vi "Rotate.vi"(2 "Angle(rad)":dbl format="%.5f", 3 "Y":dbl format="%.2f", 4 "X":dbl format="%.2f") -> (0 "rotY":dbl format="%.5f", 1 "rotX":dbl format="%.5f")   [LabVIEW 2011]
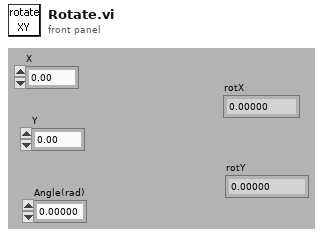
[diagram p1: front panel]
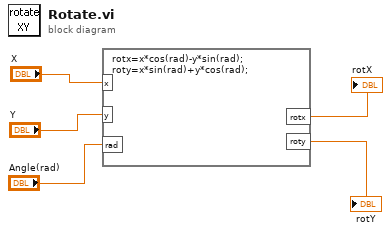
[diagram p0: block diagram]
diagram:
  n1 = formula code="rotx=x*cos(rad)-y*sin(rad);\nroty=x*sin(rad)+y*cos(rad);"("x"="X", "y"="Y", "rad"="Angle(rad)") -> ("rotx"=→"rotX":dbl, "roty"=→"rotY":dbl)
